vi "togli acq vuote.vi"(11 "Q":string[](array[string])) -> (3 "Array":string[](array[string]))   [LabVIEW 2019]
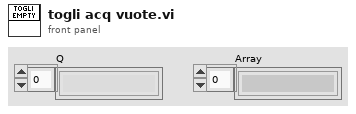
[diagram p1: front panel]
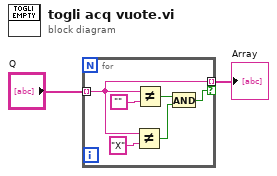
[diagram p0: block diagram]
diagram:
  n1 = for {
    tunnel: "Q" -> [w6] mode=indexing
    tunnel: [w6] -> w2 mode=indexing if=w3
    n2 = Not Equal?(x=w6, y="X") -> (x != y?=w4:bool)
    n3 = Not Equal?(x=w6, y="") -> (x != y?=w7:bool)
    n4 = And(x=w7, y=w4) -> (x .and. y?=w3:bool)
  }
  "Array" <- w2
